vi "Untitled 5.vi"() -> ()   [LabVIEW 2012]
panel:
  out "Numeric 4":i32
  in  "Numeric 3":i32
  out "Numeric 2":i32
  in  "Numeric":i32
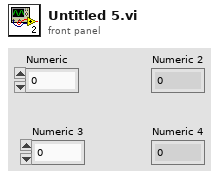
[diagram p1: front panel]
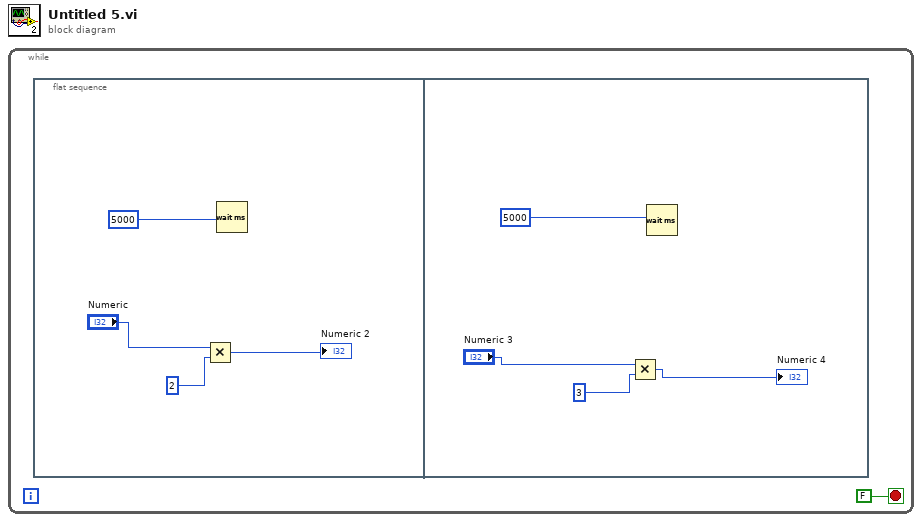
[diagram p0: block diagram]
diagram:
  n1 = while {
    stop <- FALSE stop-if-true
    n2 = flat-sequence {
      frame #0 {
        n3 = Multiply(x="Numeric", y=2) -> (x*y=→"Numeric 2":i32)
        n4 = Wait (ms)(milliseconds to wait=5000) -> ()  [unwired: 1 out]
      }
      frame #1 {
        n5 = Multiply(x="Numeric 3", y=3) -> (x*y=→"Numeric 4":i32)
        n6 = Wait (ms)(milliseconds to wait=5000) -> ()  [unwired: 1 out]
      }
    }
  }
